vi "LSCI332WriteCalFile.vi"(0 "Start path":path=path "" caption="Répertoire Initiale", 1 "Nom":string="CourbeTest", 2 "No Courbe":u32=21 min=21 max=60 step=1, 5 "No de série":string="Standard", 7 "Coefficient":u16(ring)=2 items=["Faites un choix", "négatif", "positif"], 9 "Format":u16(ring)=2 items=["Faites un choix", "mV/K", "V/K", "Ohm/K", "log Ohm/K", "log Ohm/log K"], 11 "error in":errorcluster, 12 "TLim":dbl=475.0 caption="T° de Contrôle Max (K)", 13 "Table":string[][](table)=[["7.9330000E-2", "4.8000000E+2"], ["9.0620000E-2", "4.7500000E+2"], ["1.0191000E-1", "4.7000000E+2"], ["1.1356000E-1", "4.6500000E+2"], ["1.2547000E-1", "4.6000000E+2"], ["1.3759000E-1", "4.5500000E+2"], ["1.4985000E-1", "4.5000000E+2"], ["1.6221000E-1", "4.4500000E+2"], ["1.7464000E-1", "4.4000000E+2"], ["1.8710000E-1", "4.3500000E+2"], ["1.9961000E-1", "4.3000000E+2"], ["2.2463000E-1", "4.2000000E+2"], ["2.4964000E-1", "4.1000000E+2"], ["2.7456000E-1", "4.0000000E+2"], ["2.8701000E-1", "3.9500000E+2"], ["3.2417000E-1", "3.8000000E+2"], ["3.6111000E-1", "3.6500000E+2"], ["4.1005000E-1", "3.4500000E+2"], ["4.4647000E-1", "3.3000000E+2"], ["4.5860000E-1", "3.2500000E+2"], ["5.0691000E-1", "3.0500000E+2"], ["5.1892000E-1", "3.0000000E+2"], ["5.5494000E-1", "2.8500000E+2"], ["6.0275000E-1", "2.6500000E+2"], ["6.3842000E-1", "2.5000000E+2"], ["6.7389000E-1", "2.3500000E+2"], ["7.0909000E-1", "2.2000000E+2"], ["7.4400000E-1", "2.0500000E+2"], ["7.7857000E-1", "1.9000000E+2"], ["8.0139000E-1", "1.8000000E+2"], ["8.2405000E-1", "1.7000000E+2"], ["8.4651000E-1", "1.6000000E+2"], ["8.6874000E-1", "1.5000000E+2"], ["8.7976000E-1", "1.4500000E+2"], ["8.9072000E-1", "1.4000000E+2"], ["9.0161000E-1", "1.3500000E+2"], ["9.1243000E-1", "1.3000000E+2"], ["9.2317000E-1", "1.2500000E+2"], ["9.3383000E-1", "1.2000000E+2"], ["9.4440000E-1", "1.1500000E+2"], ["9.5487000E-1", "1.1000000E+2"], ["9.6524000E-1", "1.0500000E+2"], ["9.7550000E-1", "1.0000000E+2"], ["9.8564000E-1", "9.5000000E+1"], ["9.9565000E-1", "9.0000000E+1"], ["1.0055200E+0", "8.5000000E+1"], ["1.0152500E+0", "8.0000000E+1"], ["1.0248200E+0", "7.5000000E+1"], ["1.0342500E+0", "7.0000000E+1"], ["1.0435300E+0", "6.5000000E+1"], ["1.0563000E+0", "5.8000000E+1"], ["1.0670200E+0", "5.2000000E+1"], ["1.0775000E+0", "4.6000000E+1"], ["1.0878100E+0", "4.0000000E+1"], ["1.0895300E+0", "3.9000000E+1"], ["1.0948900E+0", "3.6000000E+1"], ["1.0986400E+0", "3.4000000E+1"], ["1.1006000E+0", "3.3000000E+1"], ["1.1026300E+0", "3.2000000E+1"], ["1.1047600E+0", "3.1000000E+1"], ["1.1070200E+0", "3.0000000E+1"], ["1.1094500E+0", "2.9000000E+1"], ["1.1121200E+0", "2.8000000E+1"], ["1.1151700E+0", "2.7000000E+1"], ["1.1189600E+0", "2.6000000E+1"], ["1.1246300E+0", "2.5000000E+1"], ["1.1359800E+0", "2.4000000E+1"], ["1.1555800E+0", "2.3000000E+1"], ["1.1770500E+0", "2.2000000E+1"], ["1.1964500E+0", "2.1000000E+1"], ["1.2232100E+0", "1.9500000E+1"], ["1.2668500E+0", "1.7000000E+1"], ["1.3040400E+0", "1.5000000E+1"], ["1.3343800E+0", "1.3500000E+1"], ["1.3564200E+0", "1.2500000E+1"], ["1.3801200E+0", "1.1500000E+1"], ["1.4060500E+0", "1.0500000E+1"], ["1.4347400E+0", "9.5000000E+0"], ["1.4668400E+0", "8.5000000E+0"], ["1.5025800E+0", "7.5000000E+0"], ["1.5907500E+0", "5.2000000E+0"], ["1.6262200E+0", "4.2000000E+0"], ["1.6515600E+0", "3.4000000E+0"], ["1.6739800E+0", "2.6000000E+0"], ["1.6858500E+0", "2.1000000E+0"], ["1.6936700E+0", "1.7000000E+0"], ["1.6981800E+0", "1.4000000E+0"], ["1.7041900E+0", "1.0000000E+0"], ["0.0000000E+0", "0.0000000E+0"]] caption="Table de Calibration") -> (15 "error out":errorcluster)   [LabVIEW 2019]
doc: "Ce Vi écrit l'entête et les points d'une courbe de calibration dans un fichier texte et le sauvegarde sur le disque."
panel:
  # "+5"
  # "+10"
  # "+15"
  # "+20"
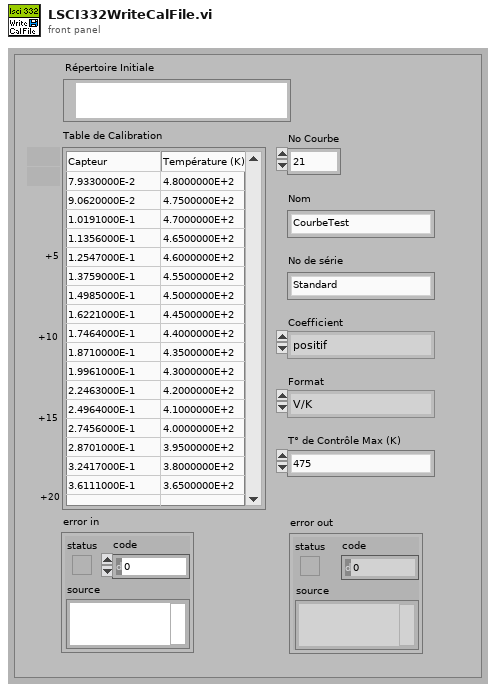
[diagram p1: front panel]
types:
  T1 = enum16{"open", "open or create", "create or replace", "create", "open (read only)"}
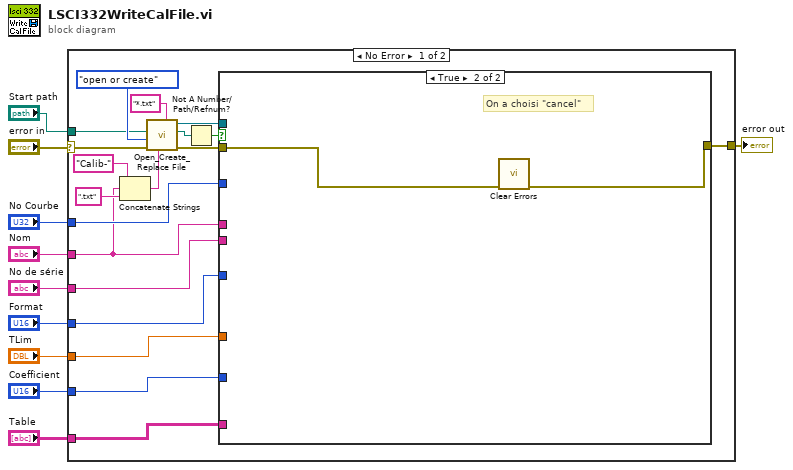
[diagram p0: block diagram]
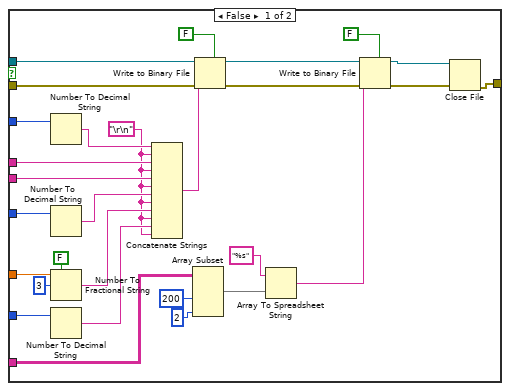
[diagram p2: hidden frame]
diagram:
  n1 = case shown="No Error" "error in" {
    selector: "error in" -> [w27 w61]
    tunnel: [w26 w61] -> w9
    tunnel: "No Courbe" -> [w23 _]
    tunnel: "Format" -> [w22 _]
    tunnel: "No de série" -> [w18 _]
    tunnel: "TLim" -> [w21 _]
    tunnel: "Coefficient" -> [w20 _]
    tunnel: "Table" -> [w19 _]
    tunnel: "Nom" -> [w11 _]
    tunnel: "Start path" -> [w16 _]
    frame No Error {
      n2 = Concatenate Strings("Calib-", w11, ".txt") -> (w12:string)
      n3 = call <vilib>:"Open_Create_Replace File.vi"("pattern"="*.txt", "default name"=w12, "error in (no error)"=w27, "function (open:0)"=T1."open or create", "start path  (Not A Path)"=w16) -> ("error out"=w28:errorcluster, "new file path"=w25:path, "refnum"=w29:refnum<file>)  [unwired: 3 in, 1 out]
      n4 = Not A Number/Path/Refnum?(number/path/refnum=w25) -> (NaN/Path/Refnum?=w24:bool)
      n5 = case shown="True" w24 {
        tunnel: w29 -> [w41 _]
        tunnel: w28 -> [w40 w60]
        tunnel: [w58 w59] -> w26
        tunnel: w23 -> [w57 _]
        tunnel: w22 -> [w56 _]
        tunnel: w21 -> [w53 _]
        tunnel: w20 -> [w52 _]
        tunnel: w19 -> [w38 _]
        tunnel: w18 -> [w46 _]
        tunnel: w11 -> [w47 _]
        frame False {
          w42 = "\r\n"
          n6 = Number To Decimal String(number=w57) -> (decimal integer string=w48:string)  [unwired: 1 in]
          n7 = Number To Decimal String(number=w56) -> (decimal integer string=w45:string)  [unwired: 1 in]
          n8 = Number To Fractional String(use system decimal point (T)=FALSE, number=w53, width (-)=3) -> (F-format string=w44:string)  [unwired: 1 in]
          n9 = Number To Decimal String(number=w52) -> (decimal integer string=w43:string)  [unwired: 1 in]
          n10 = Concatenate Strings(w48, w42, w47, w42, w46, w42, w45, w42, w44, w42, w43, w42) -> (w32:string)
          n11 = Array Subset(array=w38, length (row)=200, length (col)=2) -> (w49:string[][])  [unwired: 2 in]
          n12 = Write to Binary File(file (use dialog)=w41, data=w32, error in=w40, 5:FALSE ("ajouter une taille de tableau ou de chaîne ? (V)")) -> (refnum out=w37:refnum<file>, error out=w36:errorcluster)  [unwired: 2 in, 1 out]
          n13 = Array To Spreadsheet String(array=w49, 3:"%s") -> (spreadsheet string=w33:string)  [unwired: 1 in]
          n14 = Write to Binary File(file (use dialog)=w37, data=w33, error in=w36, 5:FALSE ("ajouter une taille de tableau ou de chaîne ? (V)")) -> (refnum out=w34:refnum<file>, error out=w35:errorcluster)  [unwired: 2 in, 1 out]
          n15 = Close File(refnum=w34, error in=w35) -> (error out=w58:errorcluster)  [unwired: 1 out]
        }
        frame True {
          # "On a choisi \"cancel\""
          n16 = call <vilib>:"Clear Errors.vi"("error in (no error)"=w60) -> ("error out"=w59:errorcluster)  [unwired: 5 in, 1 out]
        }
      }
    }
    frame Error {
    }
  }
  "error out" <- w9
